vi "scaler1.vi"(11 "L_k(t)":ext[][](array[numeric])) -> (3 "L_k(t)":ext[][](array[numeric]))   [LabVIEW 2013]
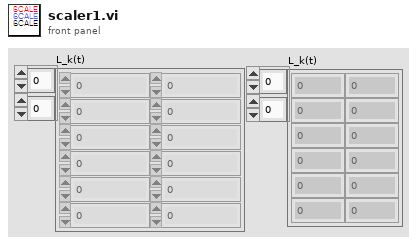
[diagram p1: front panel]
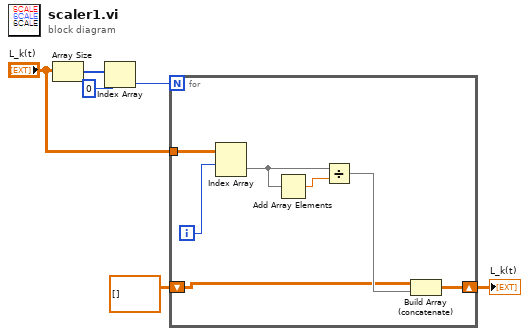
[diagram p0: block diagram]
diagram:
  n1 = Array Size(array="L_k(t)") -> (size(s)=w6:i32[])
  n2 = Index Array(array=w6, index=0) -> (element=w5:i32)
  n3 = for {
    N: w5 -> [_]
    tunnel: "L_k(t)" -> [w13]
    shift-right: [w8] -> w1
    shift-left: dbl[][] [] -> [w7]
    i -> [w12]
    n4 = Index Array(array=w13, index (row)=w12) -> (element=w10:ext[])  [unwired: 1 in]
    n5 = Add Array Elements(numeric array=w10) -> (sum=w11:ext)
    n6 = Divide(x=w10, y=w11) -> (x/y=w9:ext[])
    n7 = Build Array (concatenate)(w7, w9) -> (w8:ext[][])
  }
  "L_k(t)" <- w1
